vi "GetDgain.vi"(0 "Handle":u32, 1 "Controller Channel":i32) -> (7 "FT_Status":u32(ring) items=["FT_OK", "FT_INVALID_HANDLE", "FT_DEVICE_NOT_FOUND", "FT_DEVICE_NOT_OPENED", "FT_IO_ERROR", "FT_INSUFFICIENT_RESOURCES", "FT_INVALID_PARAMETER", "FT_INVALID_BAUD_RATE", "FT_DEVICE_NOT_OPENED_FOR_ERASE", "FT_DEVICE_NOT_OPENED_FOR_WRITE", "FT_FAILED_TO_WRITE_DEVICE", "FT_EEPROM_READ_FAILED", "FT_EEPROM_WRITE_FAILED", "FT_EEPROM_ERASE_FAILED", "FT_EEPROM_NOT_PRESENT", "FT_EEPROM_NOT_PROGRAMMED", "FT_INVALID_ARGS", "FT_NOT_SUPPORTED", "FT_OTHER_ERROR"], 9 "Dgain":dbl)   [LabVIEW 2011]
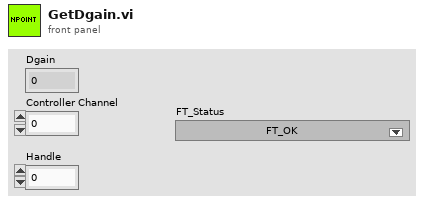
[diagram p1: front panel]
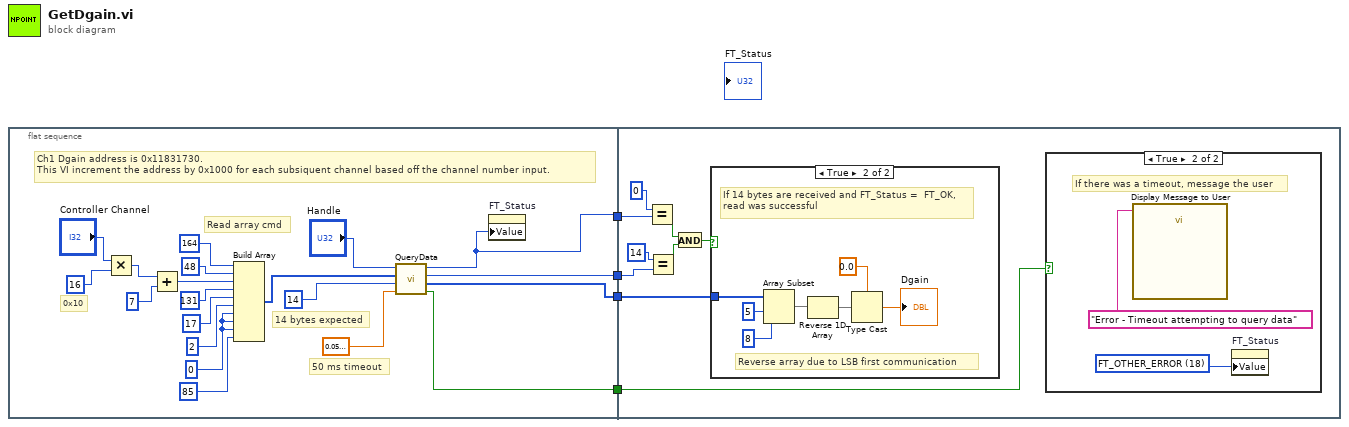
[diagram p0: block diagram]
diagram:
  n1 = flat-sequence {
    tunnel: [w11] -> w4
    tunnel: [w10] -> w3
    tunnel: [w9] -> w2
    tunnel: [w8] -> w1
    tunnel: w4 -> [w33]
    tunnel: w3 -> [w31]
    tunnel: w2 -> [w30]
    tunnel: w1 -> [w28]
    frame #0 {
      w6 = u8 0 ("element")
      # "Read array cmd"
      # "14 bytes expected"
      # "50 ms timeout"
      # "Ch1 Dgain address is 0x11831730.\nThis VI increment the address by 0x1000 for each subsiquent channel based off the channel number input."
      # "0x10"
      n2 = Multiply(x="Controller Channel", y=u8 16) -> (x*y=w17:i32)
      n3 = Add(x=w17, y=u8 7 ("element")) -> (x+y=w16:i32)
      n4 = Build Array(u8 164 ("element"), u8 48 ("element"), w16, u8 131 ("element"), u8 17 ("element"), u8 2 ("element"), w6, w6, w6, u8 85 ("element")) -> (w14:i32[])
      n5 = call "QueryData.vi"("TimeoutLengthSeconds"=sgl 0.05, "NumBytesExpected"=u32 14, "Message"=w14, "Handle"="Handle") -> ("Timeout"=w9:bool, "Return Array"=w10:u8[], "Bytes Read"=w11:u32, "FT_Status"=w8:u32)  [unwired: 4 in]
      n6 = property on="FT_Status" class="Ring (strict)"("Value"=w8) -> ()  [unwired: 2 in, 2 out]
    }
    frame #1 {
      n7 = Equal?(x=u32 0, y=w28) -> (x = y?=w26:bool)
      n8 = Equal?(x=u32 14, y=w33) -> (x = y?=w27:bool)
      n9 = And(x=w26, y=w27) -> (x .and. y?=w25:bool)
      n10 = case shown="True" w25 {
        tunnel: w31 -> [_ w42]
        frame False {
        }
        frame True {
          # "Reverse array due to LSB first communication"
          # "If 14 bytes are received and FT_Status =  FT_OK,\nread was successful"
          n11 = Array Subset(array=w42, index=5, length=8) -> (w39:u8[])
          n12 = Reverse 1D Array(array=w39) -> (reversed array=w38:u8[])
          n13 = Type Cast(type=0.0, x=w38) -> (*(type *) &x=→"Dgain":dbl)
        }
      }
      n14 = case shown="True" w30 {
        frame False {
        }
        frame True {
          w34 = u32 18 items=["FT_OK", "FT_INVALID_HANDLE", "FT_DEVICE_NOT_FOUND", "FT_DEVICE_NOT_OPENED", "FT_IO_ERROR", "FT_INSUFFICIENT_RESOURCES", "FT_INVALID_PARAMETER", "FT_INVALID_BAUD_RATE", "FT_DEVICE_NOT_OPENED_FOR_ERASE", "FT_DEVICE_NOT_OPENED_FOR_WRITE", "FT_FAILED_TO_WRITE_DEVICE", "FT_EEPROM_READ_FAILED", "FT_EEPROM_WRITE_FAILED", "FT_EEPROM_ERASE_FAILED", "FT_EEPROM_NOT_PRESENT", "FT_EEPROM_NOT_PROGRAMMED", "FT_INVALID_ARGS", "FT_NOT_SUPPORTED", "FT_OTHER_ERROR"] ("FT_Status")
          # "If there was a timeout, message the user"
          n15 = call "Display Message to User"("Message"="Error - Timeout attempting to query data") -> ()  [unwired: 9 in, 2 out]
          n16 = property on="FT_Status" class="Ring (strict)"("Value"=w34) -> ()  [unwired: 2 in, 2 out]
        }
      }
    }
  }
